vi "WPI_CANTalonSRX_GetPID.vi"(0 "CAN Talon SRX Ref":T1={"DeviceStatus"={"status"=FALSE, "code"=0, "source"=""}, "Type"=enum."PWM", "PWM"={"PWM Channel"=enum."PWM 1", "DeadBand"={"Name"="", "maxPositivePwm"=0, "minPositivePwm"=0, "centerPwm"=0, "maxNegativePwm"=0, "minNegativePwm"=0, "angularRange"=0}}, "CAN"={"Device Number"=0, "SetOutput VI Ref"=variant(enum8{"Percent VBus", "Current", "Speed", "Position", "Voltage"} enum."Percent VBus"), "GetOutput VI Ref"=variant(refnum<k1> refnum), "Enable VI Ref"=variant(dbl 12.0), "Disable VI Ref"=variant(enum8{"Percent VBus", "Speed", "Position", "Slave", "Unchanged / Invalid", "Voltage Compensation", "Current", "Motion Profile"} enum."Percent VBus"), "Data"=variant}, "Invert"=FALSE}, 1 "Parameter Slot":u8 max=1, 11 "error in (no error)":errorcluster) -> (4 "CAN Talon SRX Ref":T1={"DeviceStatus"={"status"=FALSE, "code"=0, "source"=""}, "Type"=enum."PWM", "PWM"={"PWM Channel"=enum."PWM 1", "DeadBand"={"Name"="", "maxPositivePwm"=0, "minPositivePwm"=0, "centerPwm"=0, "maxNegativePwm"=0, "minNegativePwm"=0, "angularRange"=0}}, "CAN"={"Device Number"=0, "SetOutput VI Ref"=variant(enum8{"Percent VBus", "Current", "Speed", "Position", "Voltage"} enum."Percent VBus"), "GetOutput VI Ref"=variant(refnum<k1> refnum), "Enable VI Ref"=variant(dbl 12.0), "Disable VI Ref"=variant(enum8{"Percent VBus", "Speed", "Position", "Slave", "Unchanged / Invalid", "Voltage Compensation", "Current", "Motion Profile"} enum."Percent VBus"), "Data"=variant}, "Invert"=FALSE}, 6 "P":dbl, 8 "I":dbl, 10 "D":dbl, 12 "F":dbl, 13 "I Zone":dbl, 14 "Ramp Rate":dbl, 15 "error out":errorcluster)   [LabVIEW 2016]
doc: "Get the PID constants that are being used by the active controller on the Jaguar.\n\nThis VI only applies in <B>Current</B>, <B>Position</B>, and <B>Speed</B> modes."
uses:
  <vilib>/Rock Robotics/WPI/MotorControl/WPI_MotorControlDeviceRef.ctl
  <vilib>/Rock Robotics/WPI/MotorControl/WPI_MotorControlType.ctl
  <vilib>/Rock Robotics/SystemInterfaces/DIO/FPGA_DIOPWMChannel.ctl
  <vilib>/Rock Robotics/WPI/PWM/WPI_PWMDeadband.ctl
  WPI_CANTalonSRX_MessageIDs.ctl
  WPI_CANTalonSRX_Params.ctl
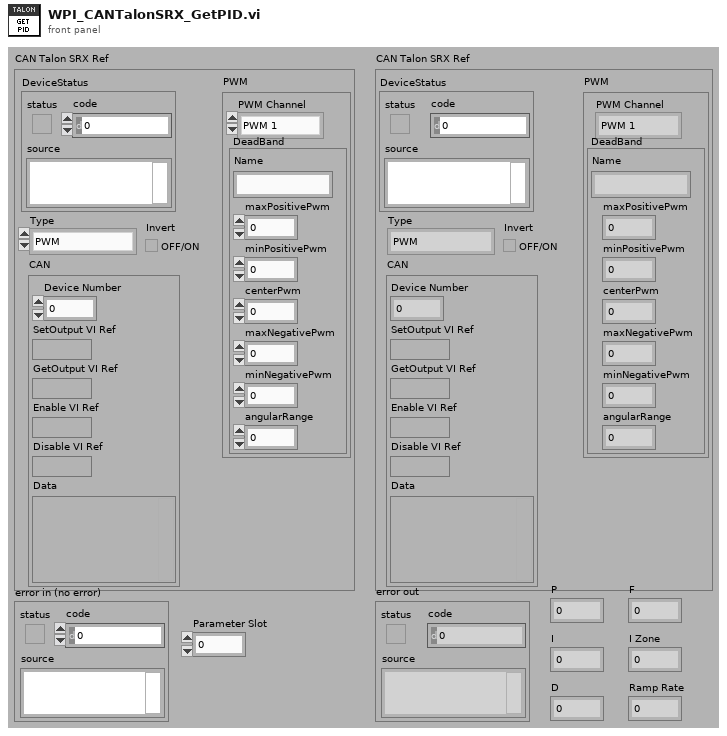
[diagram p1: front panel]
types:
  T1 = typedef "WPI_MotorControlDeviceRef.ctl" = cluster{"DeviceStatus":errorcluster, "Type":T2, "PWM":cluster{"PWM Channel":T3, "DeadBand":T4}, "CAN":cluster{"Device Number":u8, "SetOutput VI Ref":variant, "GetOutput VI Ref":variant, "Enable VI Ref":variant, "Disable VI Ref":variant, "Data":variant}, "Invert":bool}
  T2 = typedef "WPI_MotorControlType.ctl" = enum16{"PWM", "CAN"}
  T3 = typedef "FPGA_DIOPWMChannel.ctl" = enum8{"PWM 0", "PWM 1", "PWM 2", "PWM 3", "PWM 4", "PWM 5", "PWM 6", "PWM 7", "PWM 8", "PWM 9", "PWM MXP 0", "PWM MXP 1", "PWM MXP 2", "PWM MXP 3", "PWM MXP 4", "PWM MXP 5", "PWM MXP 6", "PWM MXP 7", "PWM MXP 8", "PWM MXP 9", "Invalid"}
  T4 = typedef "WPI_PWMDeadband.ctl" = cluster{"Name":string, "maxPositivePwm":i32, "minPositivePwm":i32, "centerPwm":i32, "maxNegativePwm":i32, "minNegativePwm":i32, "angularRange":u16}
  T5 = typedef "WPI_CANTalonSRX_MessageIDs.ctl" = u32
  T6 = cluster{"Message ID":u32, "Timestamp":u32, "Data":u8[]}[]
  T7 = typedef "WPI_CANTalonSRX_Params.ctl" = u8
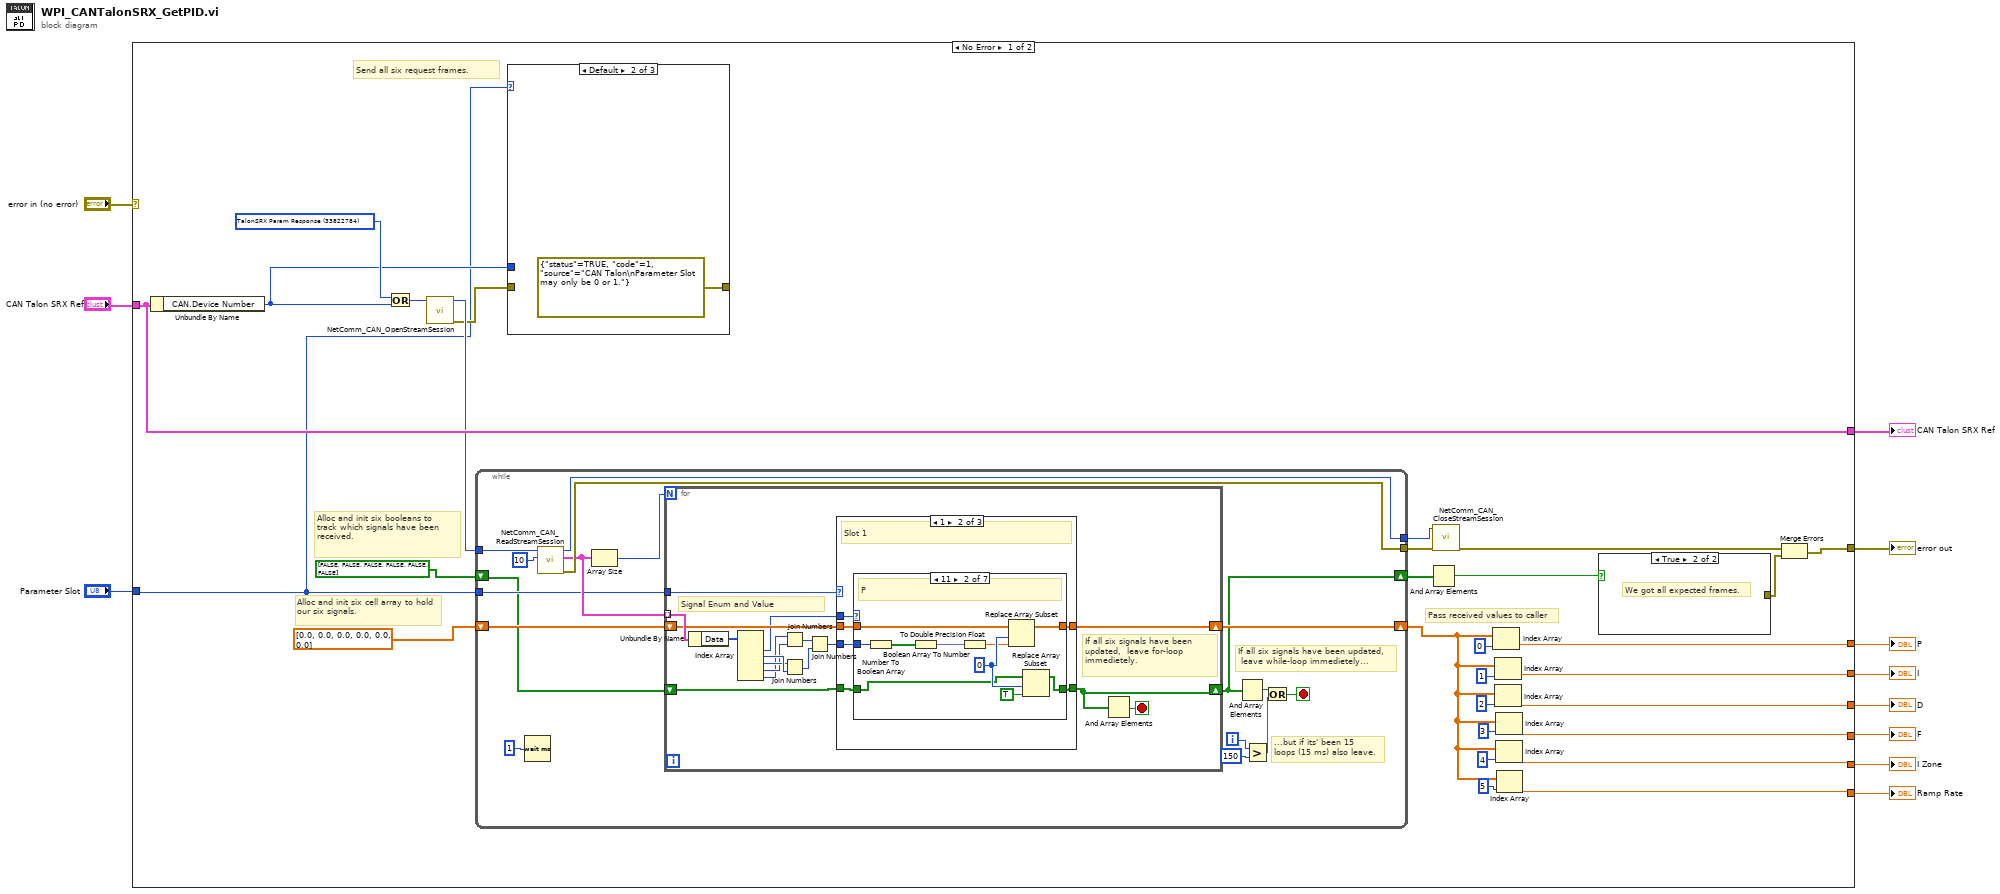
[diagram p0: block diagram]
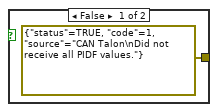
[diagram p2: hidden frame]
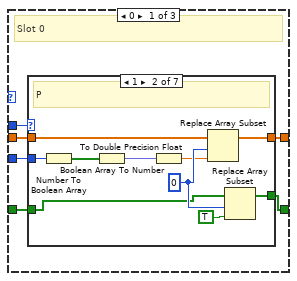
[diagram p3: hidden frame]
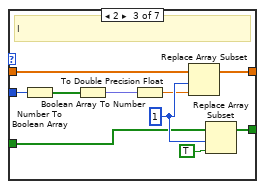
[diagram p5: hidden frame]
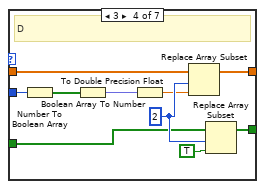
[diagram p6: hidden frame]
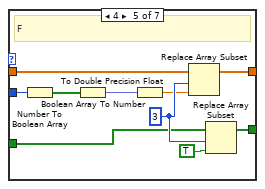
[diagram p7: hidden frame]
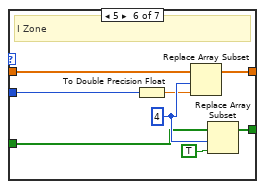
[diagram p8: hidden frame]
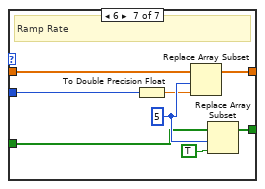
[diagram p9: hidden frame]
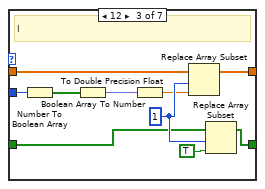
[diagram p11: hidden frame]
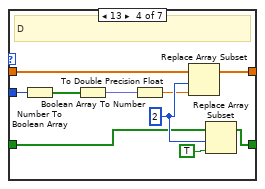
[diagram p12: hidden frame]
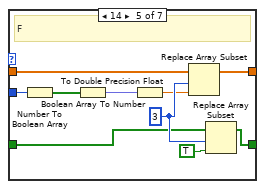
[diagram p13: hidden frame]
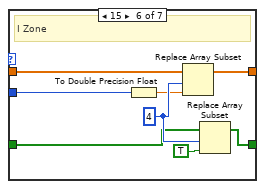
[diagram p14: hidden frame]
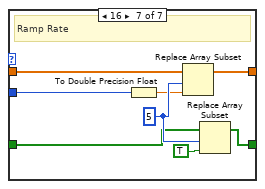
[diagram p15: hidden frame]
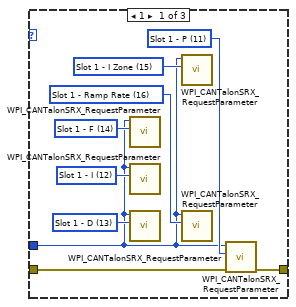
[diagram p17: hidden frame]
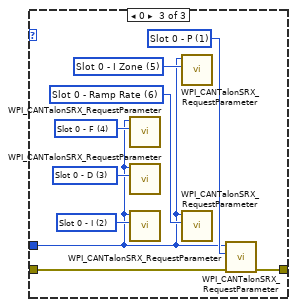
[diagram p18: hidden frame]
diagram:
  n1 = case shown="No Error" "error in (no error)" {
    selector: "error in (no error)" -> [_ w224]
    tunnel: [w40 w225] -> w11
    tunnel: "CAN Talon SRX Ref" -> [w40 w225]
    tunnel: [w15 w224] -> w9
    tunnel: "Parameter Slot" -> [w32 _]
    tunnel: [w30 _] -> w6
    tunnel: [w19 _] -> w5
    tunnel: [w24 _] -> w4
    tunnel: [w23 _] -> w3
    tunnel: [w22 _] -> w2
    tunnel: [w21 _] -> w1
    frame No Error {
      w39 = T5 33822784 items=["TalonSRX Control General 10ms"=33816576, "TalonSRX Control Rates Slow"=33816640, "TalonSRX Control ClearFlags Slow"=33816704, "TalonSRX Status General 10ms"=33821696, "TalonSRX Status Feedback 20ms"=33821760, "TalonSRX Status Enc 100ms"=33821824, "TalonSRX Status AinTempVbat 100ms"=33821888, "TalonSRX Status Startup Once"=33821952, "TalonSRX Status Debug"=33822080, "TalonSRX Config SetGainsSlot0 A"=33823808, "TalonSRX Config SetGainsSlot0 B"=33823872, "TalonSRX Config SetGainsSlot1 A"=33823936, "TalonSRX Config SetGainsSlot1 B"=33824000, "TalonSRX Config SetSoftLimits"=33824064, "TalonSRX Config WebControl"=33824128, "TalonSRX Param Request"=33822720, "TalonSRX Param Response"=33822784, "TalonSRX Param Set"=33822848]
      # "Pass received values to caller"
      # "Send all six request frames."
      # "Alloc and init six booleans to track which signals have been received."
      # "Alloc and init six cell array to hold our six signals."
      n2 = Unbundle By Name(w40) -> ("CAN.Device Number"=w38:u8)
      n3 = Or(x=w39, y=w38) -> (x .or. y?=w37:T5)
      n4 = call <vilib>:"NetComm_CAN_OpenStreamSession.vi"("Message ID"=w37) -> ("error out"=w33:errorcluster, "Session Handle"=w36:u32)  [unwired: 9 in]
      n5 = while {
        tunnel: [w55] -> w34
        tunnel: w36 -> [w58]
        tunnel: [w56] -> w35
        tunnel: w32 -> [w44]
        shift-right: [w47] -> w20
        shift-left: dbl[] [0.0, 0.0, 0.0, 0.0, 0.0, 0.0] ("Array") -> [w43]
        shift-right: [w45] -> w14
        shift-left: bool[] [FALSE, FALSE, FALSE, FALSE, FALSE, FALSE] ("Array") -> [w42]
        i -> [w53]
        stop <- w54 stop-if-true
        # "If all six signals have been updated,\n leave while-loop immedietely..."
        # "...but if its' been 15 \nloops (15 ms) also leave."
        n6 = Wait (ms)(milliseconds to wait=u32 1) -> ()  [unwired: 1 out]
        n7 = call <vilib>:"NetComm_CAN_ReadStreamSession.vi"("Messages To Read"=u32 10, "Session Handle"=w58) -> ("error out"=w55:errorcluster, "Messages"=w49:T6, "Session Handle Out"=w56:u32)  [unwired: 7 in]
        n8 = Array Size(array=w49) -> (size(s)=w46:i32)
        n9 = for {
          N: w46 -> [_]
          tunnel: w49 -> [w74] mode=indexing
          shift-right: [w62] -> w47
          shift-left: w43 -> [w64]
          shift-right: [w61] -> w45
          shift-left: w42 -> [w63]
          tunnel: w44 -> [w65]
          stop <- w66 stop-if-true
          # "Signal Enum and Value"
          # "If all six signals have been updated,  leave for-loop immedietely."
          n10 = Unbundle By Name(w74) -> ("Data"=w73:u8[])
          n11 = Index Array(array=w73) -> (element #1=w60:u8, element #2=w72:u8, element #3=w71:u8, element #4=w68:u8, element #5=w67:u8)  [unwired: 5 in]
          n12 = Join Numbers(hi=w67, lo=w68) -> ((hi.lo)=w69:u16)
          n13 = Join Numbers(hi=w71, lo=w72) -> ((hi.lo)=w70:u16)
          n14 = Join Numbers(hi=w69, lo=w70) -> ((hi.lo)=w59:u32)
          n15 = case shown="1" w65 {
            tunnel: w64 -> [w78 w144 w204]
            tunnel: w63 -> [w77 w143 w203]
            tunnel: [w75 w142 w204] -> w62
            tunnel: [w76 w141 w203] -> w61
            tunnel: w60 -> [w79 w140 _]
            tunnel: w59 -> [w80 w139 _]
            frame 0 {
              # "Slot 0"
              n16 = case shown="1" w79 {
                tunnel: [w82 w90 w97 w107 w117 w128 w134] -> w75
                tunnel: [w81 w87 w96 w106 w116 w126 w135] -> w76
                tunnel: w80 -> [_ w85 w93 w105 w115 w123 w131]
                tunnel: w78 -> [w82 w84 w95 w104 w114 w125 w132]
                tunnel: w77 -> [w81 w83 w94 w103 w113 w124 w133]
                frame Default {
                  # "Signal we don't care for"
                }
                frame 1 {
                  w88 = 0 ("index")
                  # "P"
                  n17 = Number To Boolean Array(number=w85) -> (Boolean array=w92:bool[])
                  n18 = Boolean Array To Number(Boolean array=w92) -> (number=w91:fxp<+,32,10>)
                  n19 = To Double Precision Float(number=w91) -> (double precision float=w86:dbl)
                  n20 = Replace Array Subset(array=w84, new element=w86, index=w88) -> (w90:dbl[])
                  n21 = Replace Array Subset(array=w83, new element=TRUE, index=w88) -> (w87:bool[])
                }
                frame 2 {
                  w99 = 1 ("index")
                  # "I"
                  n22 = Number To Boolean Array(number=w93) -> (Boolean array=w102:bool[])
                  n23 = Boolean Array To Number(Boolean array=w102) -> (number=w101:fxp<+,32,10>)
                  n24 = To Double Precision Float(number=w101) -> (double precision float=w98:dbl)
                  n25 = Replace Array Subset(array=w95, new element=w98, index=w99) -> (w97:dbl[])
                  n26 = Replace Array Subset(array=w94, new element=TRUE, index=w99) -> (w96:bool[])
                }
                frame 3 {
                  w109 = 2 ("index")
                  # "D"
                  n27 = Number To Boolean Array(number=w105) -> (Boolean array=w112:bool[])
                  n28 = Boolean Array To Number(Boolean array=w112) -> (number=w111:fxp<+,32,10>)
                  n29 = To Double Precision Float(number=w111) -> (double precision float=w108:dbl)
                  n30 = Replace Array Subset(array=w104, new element=w108, index=w109) -> (w107:dbl[])
                  n31 = Replace Array Subset(array=w103, new element=TRUE, index=w109) -> (w106:bool[])
                }
                frame 4 {
                  w119 = 3 ("index")
                  # "F"
                  n32 = Number To Boolean Array(number=w115) -> (Boolean array=w122:bool[])
                  n33 = Boolean Array To Number(Boolean array=w122) -> (number=w121:fxp<+/-,32,10>)
                  n34 = To Double Precision Float(number=w121) -> (double precision float=w118:dbl)
                  n35 = Replace Array Subset(array=w114, new element=w118, index=w119) -> (w117:dbl[])
                  n36 = Replace Array Subset(array=w113, new element=TRUE, index=w119) -> (w116:bool[])
                }
                frame 5 {
                  w129 = 4 ("index")
                  # "I Zone"
                  n37 = To Double Precision Float(number=w123) -> (double precision float=w127:dbl)
                  n38 = Replace Array Subset(array=w125, new element=w127, index=w129) -> (w128:dbl[])
                  n39 = Replace Array Subset(array=w124, new element=TRUE, index=w129) -> (w126:bool[])
                }
                frame 6 {
                  w137 = 5 ("index")
                  # "Ramp Rate"
                  n40 = To Double Precision Float(number=w131) -> (double precision float=w136:dbl)
                  n41 = Replace Array Subset(array=w132, new element=w136, index=w137) -> (w134:dbl[])
                  n42 = Replace Array Subset(array=w133, new element=TRUE, index=w137) -> (w135:bool[])
                }
              }
            }
            frame 1 {
              # "Slot 1"
              n43 = case shown="11" w140 {
                tunnel: w139 -> [_ w156 w166 w176 w186 w194 w202]
                tunnel: w144 -> [w145 w153 w160 w167 w179 w189 w198]
                tunnel: [w145 w152 w159 w170 w180 w191 w195] -> w142
                tunnel: w143 -> [w146 w149 w157 w168 w178 w188 w197]
                tunnel: [w146 w148 w158 w169 w177 w187 w196] -> w141
                frame Default {
                  # "Signal we don't care for"
                }
                frame 11 {
                  w150 = 0 ("index")
                  # "P"
                  n44 = Number To Boolean Array(number=w156) -> (Boolean array=w155:bool[])
                  n45 = Boolean Array To Number(Boolean array=w155) -> (number=w154:fxp<+,32,10>)
                  n46 = To Double Precision Float(number=w154) -> (double precision float=w147:dbl)
                  n47 = Replace Array Subset(array=w153, new element=w147, index=w150) -> (w152:dbl[])
                  n48 = Replace Array Subset(array=w149, new element=TRUE, index=w150) -> (w148:bool[])
                }
                frame 12 {
                  w162 = 1 ("index")
                  # "I"
                  n49 = Number To Boolean Array(number=w166) -> (Boolean array=w165:bool[])
                  n50 = Boolean Array To Number(Boolean array=w165) -> (number=w164:fxp<+,32,10>)
                  n51 = To Double Precision Float(number=w164) -> (double precision float=w161:dbl)
                  n52 = Replace Array Subset(array=w160, new element=w161, index=w162) -> (w159:dbl[])
                  n53 = Replace Array Subset(array=w157, new element=TRUE, index=w162) -> (w158:bool[])
                }
                frame 13 {
                  w172 = 2 ("index")
                  # "D"
                  n54 = Number To Boolean Array(number=w176) -> (Boolean array=w175:bool[])
                  n55 = Boolean Array To Number(Boolean array=w175) -> (number=w174:fxp<+,32,10>)
                  n56 = To Double Precision Float(number=w174) -> (double precision float=w171:dbl)
                  n57 = Replace Array Subset(array=w167, new element=w171, index=w172) -> (w170:dbl[])
                  n58 = Replace Array Subset(array=w168, new element=TRUE, index=w172) -> (w169:bool[])
                }
                frame 14 {
                  w182 = 3 ("index")
                  # "F"
                  n59 = Number To Boolean Array(number=w186) -> (Boolean array=w185:bool[])
                  n60 = Boolean Array To Number(Boolean array=w185) -> (number=w184:fxp<+/-,32,10>)
                  n61 = To Double Precision Float(number=w184) -> (double precision float=w181:dbl)
                  n62 = Replace Array Subset(array=w179, new element=w181, index=w182) -> (w180:dbl[])
                  n63 = Replace Array Subset(array=w178, new element=TRUE, index=w182) -> (w177:bool[])
                }
                frame 15 {
                  w192 = 4 ("index")
                  # "I Zone"
                  n64 = To Double Precision Float(number=w194) -> (double precision float=w190:dbl)
                  n65 = Replace Array Subset(array=w189, new element=w190, index=w192) -> (w191:dbl[])
                  n66 = Replace Array Subset(array=w188, new element=TRUE, index=w192) -> (w187:bool[])
                }
                frame 16 {
                  w200 = 5 ("index")
                  # "Ramp Rate"
                  n67 = To Double Precision Float(number=w202) -> (double precision float=w199:dbl)
                  n68 = Replace Array Subset(array=w198, new element=w199, index=w200) -> (w195:dbl[])
                  n69 = Replace Array Subset(array=w197, new element=TRUE, index=w200) -> (w196:bool[])
                }
              }
            }
            frame Default {
              # "Invalid Slot"
            }
          }
          n70 = And Array Elements(Boolean array=w61) -> (logical AND=w66:bool)
        }
        n71 = And Array Elements(Boolean array=w45) -> (logical AND=w48:bool)
        n72 = Greater?(x=w53, y=150) -> (0:w50:bool)
        n73 = Or(x=w48, y=w50) -> (x .or. y?=w54:bool)
      }
      n74 = case shown="Default" w32 {
        tunnel: [w207 errorcluster {"status"=TRUE, "code"=1, "source"="CAN Talon\nParameter Slot may only be 0 or 1."} ("error out") w222] -> _
        tunnel: w38 -> [w206 _ w216]
        tunnel: w33 -> [w205 _ w215]
        frame 1 {
          w212 = T7 16 items=["Slot 0 - P"=1, "Slot 0 - I"=2, "Slot 0 - D"=3, "Slot 0 - F"=4, "Slot 0 - I Zone"=5, "Slot 0 - Ramp Rate"=6, "Slot 1 - P"=11, "Slot 1 - I"=12, "Slot 1 - D"=13, "Slot 1 - F"=14, "Slot 1 - I Zone"=15, "Slot 1 - Ramp Rate"=16, "Soft Limit - Forward"=21, "Soft Limit - Reverse"=22, "On Boot - Brake Mode"=31, "On Boot - Limit Normally Closed - Forward"=32, "On Boot - Limit Normally Closed - Reverse"=33, "On Boot - Limit Disabled - Forward"=34, "On Boot - Limit Disabled - Reverse"=35, "Fault - Over Temp"=41, "Fault - Under Voltage"=42, "Fault - Forward Limit"=43, "Fault - Reverse Limit"=44, "Fault - Hardware Failure"=45, "Fault - Forward Soft Limit"=46, "Fault - Reverse Soft Limit"=47, "Sticky Fault - Over Temp"=48, "Sticky Fault - Under Voltage"=49, "Sticky Fault - Forward Limit"=50, "Sticky Fault - Reverse Limit"=51, "Sticky Fault - Forward Soft Limit"=52, "Sticky Fault - Reverse Soft Limit"=53, "Applied Throttle"=61, "Closed-Loop Error"=62, "Select Feedback Device"=63, "Reverse Closed-Loop Output"=64, "Mode Select"=65, "Profile Slot Select"=66, "Ramp Throttle"=67, "Reverse Feedback Sensor"=68, "Limit Switch Enabled"=69, "Limit Switch Closed - Forward"=70, "Limit Switch Closed - Reverse"=71, "Sensor Position"=73, "Sensor Velocity"=74, "Current"=75, "Brake is Enabled"=76, "Encoder Position"=77, "Encoder Velocity"=78, "Encoder Index Rise Events"=79, "Encoder A Pin State"=80, "Encoder B Pin State"=81, "Encoder Index Pin State"=82, "Analog In with Overflow"=83, "Analog In Velocity"=84, "Temperature"=85, "Battery Voltage"=86, "Reset Count"=87, "Reset Flags"=88, "Firmware Version"=89, "Settings Changed"=90] ("Parameter")
          w211 = T7 15 items=["Slot 0 - P"=1, "Slot 0 - I"=2, "Slot 0 - D"=3, "Slot 0 - F"=4, "Slot 0 - I Zone"=5, "Slot 0 - Ramp Rate"=6, "Slot 1 - P"=11, "Slot 1 - I"=12, "Slot 1 - D"=13, "Slot 1 - F"=14, "Slot 1 - I Zone"=15, "Slot 1 - Ramp Rate"=16, "Soft Limit - Forward"=21, "Soft Limit - Reverse"=22, "On Boot - Brake Mode"=31, "On Boot - Limit Normally Closed - Forward"=32, "On Boot - Limit Normally Closed - Reverse"=33, "On Boot - Limit Disabled - Forward"=34, "On Boot - Limit Disabled - Reverse"=35, "Fault - Over Temp"=41, "Fault - Under Voltage"=42, "Fault - Forward Limit"=43, "Fault - Reverse Limit"=44, "Fault - Hardware Failure"=45, "Fault - Forward Soft Limit"=46, "Fault - Reverse Soft Limit"=47, "Sticky Fault - Over Temp"=48, "Sticky Fault - Under Voltage"=49, "Sticky Fault - Forward Limit"=50, "Sticky Fault - Reverse Limit"=51, "Sticky Fault - Forward Soft Limit"=52, "Sticky Fault - Reverse Soft Limit"=53, "Applied Throttle"=61, "Closed-Loop Error"=62, "Select Feedback Device"=63, "Reverse Closed-Loop Output"=64, "Mode Select"=65, "Profile Slot Select"=66, "Ramp Throttle"=67, "Reverse Feedback Sensor"=68, "Limit Switch Enabled"=69, "Limit Switch Closed - Forward"=70, "Limit Switch Closed - Reverse"=71, "Sensor Position"=73, "Sensor Velocity"=74, "Current"=75, "Brake is Enabled"=76, "Encoder Position"=77, "Encoder Velocity"=78, "Encoder Index Rise Events"=79, "Encoder A Pin State"=80, "Encoder B Pin State"=81, "Encoder Index Pin State"=82, "Analog In with Overflow"=83, "Analog In Velocity"=84, "Temperature"=85, "Battery Voltage"=86, "Reset Count"=87, "Reset Flags"=88, "Firmware Version"=89, "Settings Changed"=90] ("Parameter")
          w210 = T7 14 items=["Slot 0 - P"=1, "Slot 0 - I"=2, "Slot 0 - D"=3, "Slot 0 - F"=4, "Slot 0 - I Zone"=5, "Slot 0 - Ramp Rate"=6, "Slot 1 - P"=11, "Slot 1 - I"=12, "Slot 1 - D"=13, "Slot 1 - F"=14, "Slot 1 - I Zone"=15, "Slot 1 - Ramp Rate"=16, "Soft Limit - Forward"=21, "Soft Limit - Reverse"=22, "On Boot - Brake Mode"=31, "On Boot - Limit Normally Closed - Forward"=32, "On Boot - Limit Normally Closed - Reverse"=33, "On Boot - Limit Disabled - Forward"=34, "On Boot - Limit Disabled - Reverse"=35, "Fault - Over Temp"=41, "Fault - Under Voltage"=42, "Fault - Forward Limit"=43, "Fault - Reverse Limit"=44, "Fault - Hardware Failure"=45, "Fault - Forward Soft Limit"=46, "Fault - Reverse Soft Limit"=47, "Sticky Fault - Over Temp"=48, "Sticky Fault - Under Voltage"=49, "Sticky Fault - Forward Limit"=50, "Sticky Fault - Reverse Limit"=51, "Sticky Fault - Forward Soft Limit"=52, "Sticky Fault - Reverse Soft Limit"=53, "Applied Throttle"=61, "Closed-Loop Error"=62, "Select Feedback Device"=63, "Reverse Closed-Loop Output"=64, "Mode Select"=65, "Profile Slot Select"=66, "Ramp Throttle"=67, "Reverse Feedback Sensor"=68, "Limit Switch Enabled"=69, "Limit Switch Closed - Forward"=70, "Limit Switch Closed - Reverse"=71, "Sensor Position"=73, "Sensor Velocity"=74, "Current"=75, "Brake is Enabled"=76, "Encoder Position"=77, "Encoder Velocity"=78, "Encoder Index Rise Events"=79, "Encoder A Pin State"=80, "Encoder B Pin State"=81, "Encoder Index Pin State"=82, "Analog In with Overflow"=83, "Analog In Velocity"=84, "Temperature"=85, "Battery Voltage"=86, "Reset Count"=87, "Reset Flags"=88, "Firmware Version"=89, "Settings Changed"=90] ("Parameter")
          w209 = T7 13 items=["Slot 0 - P"=1, "Slot 0 - I"=2, "Slot 0 - D"=3, "Slot 0 - F"=4, "Slot 0 - I Zone"=5, "Slot 0 - Ramp Rate"=6, "Slot 1 - P"=11, "Slot 1 - I"=12, "Slot 1 - D"=13, "Slot 1 - F"=14, "Slot 1 - I Zone"=15, "Slot 1 - Ramp Rate"=16, "Soft Limit - Forward"=21, "Soft Limit - Reverse"=22, "On Boot - Brake Mode"=31, "On Boot - Limit Normally Closed - Forward"=32, "On Boot - Limit Normally Closed - Reverse"=33, "On Boot - Limit Disabled - Forward"=34, "On Boot - Limit Disabled - Reverse"=35, "Fault - Over Temp"=41, "Fault - Under Voltage"=42, "Fault - Forward Limit"=43, "Fault - Reverse Limit"=44, "Fault - Hardware Failure"=45, "Fault - Forward Soft Limit"=46, "Fault - Reverse Soft Limit"=47, "Sticky Fault - Over Temp"=48, "Sticky Fault - Under Voltage"=49, "Sticky Fault - Forward Limit"=50, "Sticky Fault - Reverse Limit"=51, "Sticky Fault - Forward Soft Limit"=52, "Sticky Fault - Reverse Soft Limit"=53, "Applied Throttle"=61, "Closed-Loop Error"=62, "Select Feedback Device"=63, "Reverse Closed-Loop Output"=64, "Mode Select"=65, "Profile Slot Select"=66, "Ramp Throttle"=67, "Reverse Feedback Sensor"=68, "Limit Switch Enabled"=69, "Limit Switch Closed - Forward"=70, "Limit Switch Closed - Reverse"=71, "Sensor Position"=73, "Sensor Velocity"=74, "Current"=75, "Brake is Enabled"=76, "Encoder Position"=77, "Encoder Velocity"=78, "Encoder Index Rise Events"=79, "Encoder A Pin State"=80, "Encoder B Pin State"=81, "Encoder Index Pin State"=82, "Analog In with Overflow"=83, "Analog In Velocity"=84, "Temperature"=85, "Battery Voltage"=86, "Reset Count"=87, "Reset Flags"=88, "Firmware Version"=89, "Settings Changed"=90] ("Parameter")
          w208 = T7 12 items=["Slot 0 - P"=1, "Slot 0 - I"=2, "Slot 0 - D"=3, "Slot 0 - F"=4, "Slot 0 - I Zone"=5, "Slot 0 - Ramp Rate"=6, "Slot 1 - P"=11, "Slot 1 - I"=12, "Slot 1 - D"=13, "Slot 1 - F"=14, "Slot 1 - I Zone"=15, "Slot 1 - Ramp Rate"=16, "Soft Limit - Forward"=21, "Soft Limit - Reverse"=22, "On Boot - Brake Mode"=31, "On Boot - Limit Normally Closed - Forward"=32, "On Boot - Limit Normally Closed - Reverse"=33, "On Boot - Limit Disabled - Forward"=34, "On Boot - Limit Disabled - Reverse"=35, "Fault - Over Temp"=41, "Fault - Under Voltage"=42, "Fault - Forward Limit"=43, "Fault - Reverse Limit"=44, "Fault - Hardware Failure"=45, "Fault - Forward Soft Limit"=46, "Fault - Reverse Soft Limit"=47, "Sticky Fault - Over Temp"=48, "Sticky Fault - Under Voltage"=49, "Sticky Fault - Forward Limit"=50, "Sticky Fault - Reverse Limit"=51, "Sticky Fault - Forward Soft Limit"=52, "Sticky Fault - Reverse Soft Limit"=53, "Applied Throttle"=61, "Closed-Loop Error"=62, "Select Feedback Device"=63, "Reverse Closed-Loop Output"=64, "Mode Select"=65, "Profile Slot Select"=66, "Ramp Throttle"=67, "Reverse Feedback Sensor"=68, "Limit Switch Enabled"=69, "Limit Switch Closed - Forward"=70, "Limit Switch Closed - Reverse"=71, "Sensor Position"=73, "Sensor Velocity"=74, "Current"=75, "Brake is Enabled"=76, "Encoder Position"=77, "Encoder Velocity"=78, "Encoder Index Rise Events"=79, "Encoder A Pin State"=80, "Encoder B Pin State"=81, "Encoder Index Pin State"=82, "Analog In with Overflow"=83, "Analog In Velocity"=84, "Temperature"=85, "Battery Voltage"=86, "Reset Count"=87, "Reset Flags"=88, "Firmware Version"=89, "Settings Changed"=90] ("Parameter")
          w213 = T7 11 items=["Slot 0 - P"=1, "Slot 0 - I"=2, "Slot 0 - D"=3, "Slot 0 - F"=4, "Slot 0 - I Zone"=5, "Slot 0 - Ramp Rate"=6, "Slot 1 - P"=11, "Slot 1 - I"=12, "Slot 1 - D"=13, "Slot 1 - F"=14, "Slot 1 - I Zone"=15, "Slot 1 - Ramp Rate"=16, "Soft Limit - Forward"=21, "Soft Limit - Reverse"=22, "On Boot - Brake Mode"=31, "On Boot - Limit Normally Closed - Forward"=32, "On Boot - Limit Normally Closed - Reverse"=33, "On Boot - Limit Disabled - Forward"=34, "On Boot - Limit Disabled - Reverse"=35, "Fault - Over Temp"=41, "Fault - Under Voltage"=42, "Fault - Forward Limit"=43, "Fault - Reverse Limit"=44, "Fault - Hardware Failure"=45, "Fault - Forward Soft Limit"=46, "Fault - Reverse Soft Limit"=47, "Sticky Fault - Over Temp"=48, "Sticky Fault - Under Voltage"=49, "Sticky Fault - Forward Limit"=50, "Sticky Fault - Reverse Limit"=51, "Sticky Fault - Forward Soft Limit"=52, "Sticky Fault - Reverse Soft Limit"=53, "Applied Throttle"=61, "Closed-Loop Error"=62, "Select Feedback Device"=63, "Reverse Closed-Loop Output"=64, "Mode Select"=65, "Profile Slot Select"=66, "Ramp Throttle"=67, "Reverse Feedback Sensor"=68, "Limit Switch Enabled"=69, "Limit Switch Closed - Forward"=70, "Limit Switch Closed - Reverse"=71, "Sensor Position"=73, "Sensor Velocity"=74, "Current"=75, "Brake is Enabled"=76, "Encoder Position"=77, "Encoder Velocity"=78, "Encoder Index Rise Events"=79, "Encoder A Pin State"=80, "Encoder B Pin State"=81, "Encoder Index Pin State"=82, "Analog In with Overflow"=83, "Analog In Velocity"=84, "Temperature"=85, "Battery Voltage"=86, "Reset Count"=87, "Reset Flags"=88, "Firmware Version"=89, "Settings Changed"=90] ("Parameter")
          n75 = call "WPI_CANTalonSRX_RequestParameter.vi"("Parameter"=w210, "Device ID (0)"=w206) -> ()  [unwired: 8 in, 2 out]
          n76 = call "WPI_CANTalonSRX_RequestParameter.vi"("Parameter"=w208, "Device ID (0)"=w206) -> ()  [unwired: 8 in, 2 out]
          n77 = call "WPI_CANTalonSRX_RequestParameter.vi"("Parameter"=w209, "Device ID (0)"=w206) -> ()  [unwired: 8 in, 2 out]
          n78 = call "WPI_CANTalonSRX_RequestParameter.vi"("Parameter"=w211, "Device ID (0)"=w206) -> ()  [unwired: 8 in, 2 out]
          n79 = call "WPI_CANTalonSRX_RequestParameter.vi"("Parameter"=w212, "Device ID (0)"=w206) -> ()  [unwired: 8 in, 2 out]
          n80 = call "WPI_CANTalonSRX_RequestParameter.vi"("error in (no error)"=w205, "Parameter"=w213, "Device ID (0)"=w206) -> ("error out"=w207:errorcluster)  [unwired: 7 in, 1 out]
        }
        frame Default {
        }
        frame 0 {
          w220 = T7 6 items=["Slot 0 - P"=1, "Slot 0 - I"=2, "Slot 0 - D"=3, "Slot 0 - F"=4, "Slot 0 - I Zone"=5, "Slot 0 - Ramp Rate"=6, "Slot 1 - P"=11, "Slot 1 - I"=12, "Slot 1 - D"=13, "Slot 1 - F"=14, "Slot 1 - I Zone"=15, "Slot 1 - Ramp Rate"=16, "Soft Limit - Forward"=21, "Soft Limit - Reverse"=22, "On Boot - Brake Mode"=31, "On Boot - Limit Normally Closed - Forward"=32, "On Boot - Limit Normally Closed - Reverse"=33, "On Boot - Limit Disabled - Forward"=34, "On Boot - Limit Disabled - Reverse"=35, "Fault - Over Temp"=41, "Fault - Under Voltage"=42, "Fault - Forward Limit"=43, "Fault - Reverse Limit"=44, "Fault - Hardware Failure"=45, "Fault - Forward Soft Limit"=46, "Fault - Reverse Soft Limit"=47, "Sticky Fault - Over Temp"=48, "Sticky Fault - Under Voltage"=49, "Sticky Fault - Forward Limit"=50, "Sticky Fault - Reverse Limit"=51, "Sticky Fault - Forward Soft Limit"=52, "Sticky Fault - Reverse Soft Limit"=53, "Applied Throttle"=61, "Closed-Loop Error"=62, "Select Feedback Device"=63, "Reverse Closed-Loop Output"=64, "Mode Select"=65, "Profile Slot Select"=66, "Ramp Throttle"=67, "Reverse Feedback Sensor"=68, "Limit Switch Enabled"=69, "Limit Switch Closed - Forward"=70, "Limit Switch Closed - Reverse"=71, "Sensor Position"=73, "Sensor Velocity"=74, "Current"=75, "Brake is Enabled"=76, "Encoder Position"=77, "Encoder Velocity"=78, "Encoder Index Rise Events"=79, "Encoder A Pin State"=80, "Encoder B Pin State"=81, "Encoder Index Pin State"=82, "Analog In with Overflow"=83, "Analog In Velocity"=84, "Temperature"=85, "Battery Voltage"=86, "Reset Count"=87, "Reset Flags"=88, "Firmware Version"=89, "Settings Changed"=90] ("Parameter")
          w219 = T7 5 items=["Slot 0 - P"=1, "Slot 0 - I"=2, "Slot 0 - D"=3, "Slot 0 - F"=4, "Slot 0 - I Zone"=5, "Slot 0 - Ramp Rate"=6, "Slot 1 - P"=11, "Slot 1 - I"=12, "Slot 1 - D"=13, "Slot 1 - F"=14, "Slot 1 - I Zone"=15, "Slot 1 - Ramp Rate"=16, "Soft Limit - Forward"=21, "Soft Limit - Reverse"=22, "On Boot - Brake Mode"=31, "On Boot - Limit Normally Closed - Forward"=32, "On Boot - Limit Normally Closed - Reverse"=33, "On Boot - Limit Disabled - Forward"=34, "On Boot - Limit Disabled - Reverse"=35, "Fault - Over Temp"=41, "Fault - Under Voltage"=42, "Fault - Forward Limit"=43, "Fault - Reverse Limit"=44, "Fault - Hardware Failure"=45, "Fault - Forward Soft Limit"=46, "Fault - Reverse Soft Limit"=47, "Sticky Fault - Over Temp"=48, "Sticky Fault - Under Voltage"=49, "Sticky Fault - Forward Limit"=50, "Sticky Fault - Reverse Limit"=51, "Sticky Fault - Forward Soft Limit"=52, "Sticky Fault - Reverse Soft Limit"=53, "Applied Throttle"=61, "Closed-Loop Error"=62, "Select Feedback Device"=63, "Reverse Closed-Loop Output"=64, "Mode Select"=65, "Profile Slot Select"=66, "Ramp Throttle"=67, "Reverse Feedback Sensor"=68, "Limit Switch Enabled"=69, "Limit Switch Closed - Forward"=70, "Limit Switch Closed - Reverse"=71, "Sensor Position"=73, "Sensor Velocity"=74, "Current"=75, "Brake is Enabled"=76, "Encoder Position"=77, "Encoder Velocity"=78, "Encoder Index Rise Events"=79, "Encoder A Pin State"=80, "Encoder B Pin State"=81, "Encoder Index Pin State"=82, "Analog In with Overflow"=83, "Analog In Velocity"=84, "Temperature"=85, "Battery Voltage"=86, "Reset Count"=87, "Reset Flags"=88, "Firmware Version"=89, "Settings Changed"=90] ("Parameter")
          w218 = T7 4 items=["Slot 0 - P"=1, "Slot 0 - I"=2, "Slot 0 - D"=3, "Slot 0 - F"=4, "Slot 0 - I Zone"=5, "Slot 0 - Ramp Rate"=6, "Slot 1 - P"=11, "Slot 1 - I"=12, "Slot 1 - D"=13, "Slot 1 - F"=14, "Slot 1 - I Zone"=15, "Slot 1 - Ramp Rate"=16, "Soft Limit - Forward"=21, "Soft Limit - Reverse"=22, "On Boot - Brake Mode"=31, "On Boot - Limit Normally Closed - Forward"=32, "On Boot - Limit Normally Closed - Reverse"=33, "On Boot - Limit Disabled - Forward"=34, "On Boot - Limit Disabled - Reverse"=35, "Fault - Over Temp"=41, "Fault - Under Voltage"=42, "Fault - Forward Limit"=43, "Fault - Reverse Limit"=44, "Fault - Hardware Failure"=45, "Fault - Forward Soft Limit"=46, "Fault - Reverse Soft Limit"=47, "Sticky Fault - Over Temp"=48, "Sticky Fault - Under Voltage"=49, "Sticky Fault - Forward Limit"=50, "Sticky Fault - Reverse Limit"=51, "Sticky Fault - Forward Soft Limit"=52, "Sticky Fault - Reverse Soft Limit"=53, "Applied Throttle"=61, "Closed-Loop Error"=62, "Select Feedback Device"=63, "Reverse Closed-Loop Output"=64, "Mode Select"=65, "Profile Slot Select"=66, "Ramp Throttle"=67, "Reverse Feedback Sensor"=68, "Limit Switch Enabled"=69, "Limit Switch Closed - Forward"=70, "Limit Switch Closed - Reverse"=71, "Sensor Position"=73, "Sensor Velocity"=74, "Current"=75, "Brake is Enabled"=76, "Encoder Position"=77, "Encoder Velocity"=78, "Encoder Index Rise Events"=79, "Encoder A Pin State"=80, "Encoder B Pin State"=81, "Encoder Index Pin State"=82, "Analog In with Overflow"=83, "Analog In Velocity"=84, "Temperature"=85, "Battery Voltage"=86, "Reset Count"=87, "Reset Flags"=88, "Firmware Version"=89, "Settings Changed"=90] ("Parameter")
          w217 = T7 3 items=["Slot 0 - P"=1, "Slot 0 - I"=2, "Slot 0 - D"=3, "Slot 0 - F"=4, "Slot 0 - I Zone"=5, "Slot 0 - Ramp Rate"=6, "Slot 1 - P"=11, "Slot 1 - I"=12, "Slot 1 - D"=13, "Slot 1 - F"=14, "Slot 1 - I Zone"=15, "Slot 1 - Ramp Rate"=16, "Soft Limit - Forward"=21, "Soft Limit - Reverse"=22, "On Boot - Brake Mode"=31, "On Boot - Limit Normally Closed - Forward"=32, "On Boot - Limit Normally Closed - Reverse"=33, "On Boot - Limit Disabled - Forward"=34, "On Boot - Limit Disabled - Reverse"=35, "Fault - Over Temp"=41, "Fault - Under Voltage"=42, "Fault - Forward Limit"=43, "Fault - Reverse Limit"=44, "Fault - Hardware Failure"=45, "Fault - Forward Soft Limit"=46, "Fault - Reverse Soft Limit"=47, "Sticky Fault - Over Temp"=48, "Sticky Fault - Under Voltage"=49, "Sticky Fault - Forward Limit"=50, "Sticky Fault - Reverse Limit"=51, "Sticky Fault - Forward Soft Limit"=52, "Sticky Fault - Reverse Soft Limit"=53, "Applied Throttle"=61, "Closed-Loop Error"=62, "Select Feedback Device"=63, "Reverse Closed-Loop Output"=64, "Mode Select"=65, "Profile Slot Select"=66, "Ramp Throttle"=67, "Reverse Feedback Sensor"=68, "Limit Switch Enabled"=69, "Limit Switch Closed - Forward"=70, "Limit Switch Closed - Reverse"=71, "Sensor Position"=73, "Sensor Velocity"=74, "Current"=75, "Brake is Enabled"=76, "Encoder Position"=77, "Encoder Velocity"=78, "Encoder Index Rise Events"=79, "Encoder A Pin State"=80, "Encoder B Pin State"=81, "Encoder Index Pin State"=82, "Analog In with Overflow"=83, "Analog In Velocity"=84, "Temperature"=85, "Battery Voltage"=86, "Reset Count"=87, "Reset Flags"=88, "Firmware Version"=89, "Settings Changed"=90] ("Parameter")
          w221 = T7 2 items=["Slot 0 - P"=1, "Slot 0 - I"=2, "Slot 0 - D"=3, "Slot 0 - F"=4, "Slot 0 - I Zone"=5, "Slot 0 - Ramp Rate"=6, "Slot 1 - P"=11, "Slot 1 - I"=12, "Slot 1 - D"=13, "Slot 1 - F"=14, "Slot 1 - I Zone"=15, "Slot 1 - Ramp Rate"=16, "Soft Limit - Forward"=21, "Soft Limit - Reverse"=22, "On Boot - Brake Mode"=31, "On Boot - Limit Normally Closed - Forward"=32, "On Boot - Limit Normally Closed - Reverse"=33, "On Boot - Limit Disabled - Forward"=34, "On Boot - Limit Disabled - Reverse"=35, "Fault - Over Temp"=41, "Fault - Under Voltage"=42, "Fault - Forward Limit"=43, "Fault - Reverse Limit"=44, "Fault - Hardware Failure"=45, "Fault - Forward Soft Limit"=46, "Fault - Reverse Soft Limit"=47, "Sticky Fault - Over Temp"=48, "Sticky Fault - Under Voltage"=49, "Sticky Fault - Forward Limit"=50, "Sticky Fault - Reverse Limit"=51, "Sticky Fault - Forward Soft Limit"=52, "Sticky Fault - Reverse Soft Limit"=53, "Applied Throttle"=61, "Closed-Loop Error"=62, "Select Feedback Device"=63, "Reverse Closed-Loop Output"=64, "Mode Select"=65, "Profile Slot Select"=66, "Ramp Throttle"=67, "Reverse Feedback Sensor"=68, "Limit Switch Enabled"=69, "Limit Switch Closed - Forward"=70, "Limit Switch Closed - Reverse"=71, "Sensor Position"=73, "Sensor Velocity"=74, "Current"=75, "Brake is Enabled"=76, "Encoder Position"=77, "Encoder Velocity"=78, "Encoder Index Rise Events"=79, "Encoder A Pin State"=80, "Encoder B Pin State"=81, "Encoder Index Pin State"=82, "Analog In with Overflow"=83, "Analog In Velocity"=84, "Temperature"=85, "Battery Voltage"=86, "Reset Count"=87, "Reset Flags"=88, "Firmware Version"=89, "Settings Changed"=90] ("Parameter")
          w223 = T7 1 items=["Slot 0 - P"=1, "Slot 0 - I"=2, "Slot 0 - D"=3, "Slot 0 - F"=4, "Slot 0 - I Zone"=5, "Slot 0 - Ramp Rate"=6, "Slot 1 - P"=11, "Slot 1 - I"=12, "Slot 1 - D"=13, "Slot 1 - F"=14, "Slot 1 - I Zone"=15, "Slot 1 - Ramp Rate"=16, "Soft Limit - Forward"=21, "Soft Limit - Reverse"=22, "On Boot - Brake Mode"=31, "On Boot - Limit Normally Closed - Forward"=32, "On Boot - Limit Normally Closed - Reverse"=33, "On Boot - Limit Disabled - Forward"=34, "On Boot - Limit Disabled - Reverse"=35, "Fault - Over Temp"=41, "Fault - Under Voltage"=42, "Fault - Forward Limit"=43, "Fault - Reverse Limit"=44, "Fault - Hardware Failure"=45, "Fault - Forward Soft Limit"=46, "Fault - Reverse Soft Limit"=47, "Sticky Fault - Over Temp"=48, "Sticky Fault - Under Voltage"=49, "Sticky Fault - Forward Limit"=50, "Sticky Fault - Reverse Limit"=51, "Sticky Fault - Forward Soft Limit"=52, "Sticky Fault - Reverse Soft Limit"=53, "Applied Throttle"=61, "Closed-Loop Error"=62, "Select Feedback Device"=63, "Reverse Closed-Loop Output"=64, "Mode Select"=65, "Profile Slot Select"=66, "Ramp Throttle"=67, "Reverse Feedback Sensor"=68, "Limit Switch Enabled"=69, "Limit Switch Closed - Forward"=70, "Limit Switch Closed - Reverse"=71, "Sensor Position"=73, "Sensor Velocity"=74, "Current"=75, "Brake is Enabled"=76, "Encoder Position"=77, "Encoder Velocity"=78, "Encoder Index Rise Events"=79, "Encoder A Pin State"=80, "Encoder B Pin State"=81, "Encoder Index Pin State"=82, "Analog In with Overflow"=83, "Analog In Velocity"=84, "Temperature"=85, "Battery Voltage"=86, "Reset Count"=87, "Reset Flags"=88, "Firmware Version"=89, "Settings Changed"=90] ("Parameter")
          n81 = call "WPI_CANTalonSRX_RequestParameter.vi"("Parameter"=w218, "Device ID (0)"=w216) -> ()  [unwired: 8 in, 2 out]
          n82 = call "WPI_CANTalonSRX_RequestParameter.vi"("Parameter"=w217, "Device ID (0)"=w216) -> ()  [unwired: 8 in, 2 out]
          n83 = call "WPI_CANTalonSRX_RequestParameter.vi"("Parameter"=w221, "Device ID (0)"=w216) -> ()  [unwired: 8 in, 2 out]
          n84 = call "WPI_CANTalonSRX_RequestParameter.vi"("Parameter"=w219, "Device ID (0)"=w216) -> ()  [unwired: 8 in, 2 out]
          n85 = call "WPI_CANTalonSRX_RequestParameter.vi"("Parameter"=w220, "Device ID (0)"=w216) -> ()  [unwired: 8 in, 2 out]
          n86 = call "WPI_CANTalonSRX_RequestParameter.vi"("error in (no error)"=w215, "Parameter"=w223, "Device ID (0)"=w216) -> ("error out"=w222:errorcluster)  [unwired: 7 in, 1 out]
        }
      }
      n87 = And Array Elements(Boolean array=w14) -> (logical AND=w13:bool)
      n88 = call <vilib>:"NetComm_CAN_CloseStreamSession.vi"("error in (no error)"=w34, "Session Handle"=w35) -> ("error out"=w16:errorcluster)  [unwired: 9 in]
      n89 = Index Array(array=w20, index=0) -> (element=w30:dbl)
      n90 = Index Array(array=w20, index=1) -> (element=w21:dbl)
      n91 = Index Array(array=w20, index=2) -> (element=w22:dbl)
      n92 = Index Array(array=w20, index=3) -> (element=w23:dbl)
      n93 = Index Array(array=w20, index=4) -> (element=w24:dbl)
      n94 = Index Array(array=w20, index=5) -> (element=w19:dbl)
      n95 = case shown="True" w13 {
        tunnel: [errorcluster {"status"=TRUE, "code"=1, "source"="CAN Talon\nDid not receive all PIDF values."} ("error out") _] -> w12
        frame False {
        }
        frame True {
          # "We got all expected frames."
        }
      }
      n96 = Merge Errors(w16, w12) -> (w15:errorcluster)
    }
    frame Error {
    }
  }
  "CAN Talon SRX Ref" <- w11
  "error out" <- w9
  "F" <- w3
  "I Zone" <- w4
  "Ramp Rate" <- w5
  "P" <- w6
  "I" <- w1
  "D" <- w2
